vi "Global_Freq.vi"() -> ()   [LabVIEW 2019]
panel:
  in  "Fs":dbl=1000.0
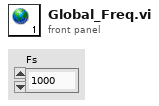
[diagram p1: front panel]
diagram:
